vi "Curvature of Bezier Curve.vi"(11 "curve":T1) -> (3 "curvature":dbl[](array[numeric]))   [LabVIEW 2019]
uses:
  Types/Bezier Curve.ctl
panel:
  in  "percision":dbl
  in  "ctrl points":cluster{dbl, dbl}[](array[cluster])
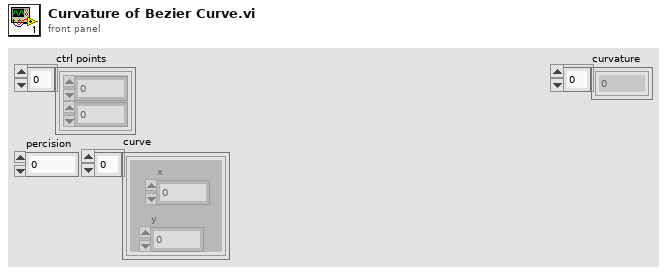
[diagram p1: front panel]
types:
  T1 = typedef "Bezier Curve.ctl" = cluster{"x":dbl, "y":dbl}[]
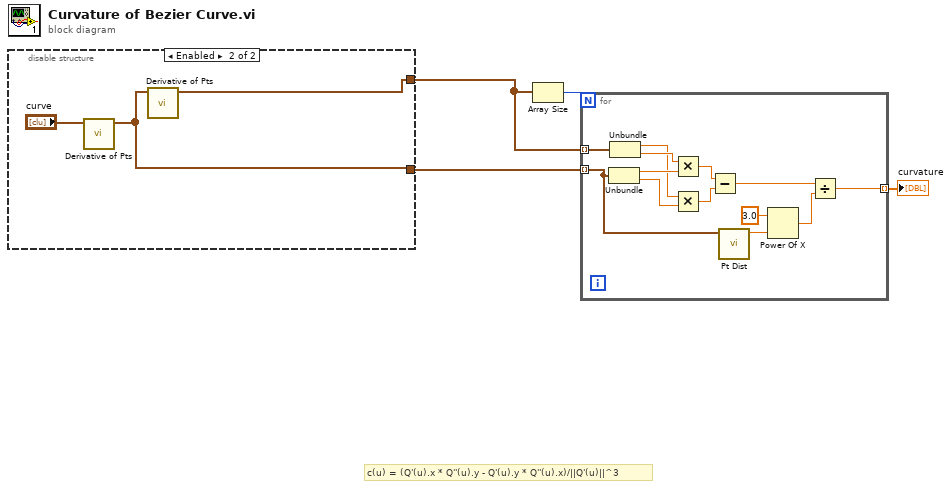
[diagram p0: block diagram]
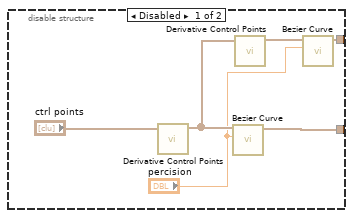
[diagram p2: hidden frame]
diagram:
  # "c(u) = (Q'(u).x * Q''(u).y - Q'(u).y * Q''(u).x)/||Q'(u)||^3"
  n1 = disable-structure shown="Enabled" {
    disable-tunnel: [w6 w12] -> w3
    disable-tunnel: [w5 w11] -> w2
    frame Disabled {
      n2 = call "Derivative Control Points.vi"("ctrl points"="ctrl points") -> ("d ctrl pts"=w9:cluster{dbl, dbl}[])  [unwired: 10 in]
      n3 = call "Bezier Curve.vi"("percision"="percision", "ctrl points"=w9) -> ("curve"=w5:T1)  [unwired: 9 in]
      n4 = call "Derivative Control Points.vi"("ctrl points"=w9) -> ("d ctrl pts"=w8:cluster{dbl, dbl}[])  [unwired: 10 in]
      n5 = call "Bezier Curve.vi"("percision"="percision", "ctrl points"=w8) -> ("curve"=w6:T1)  [unwired: 9 in]
    }
    frame Enabled {
      n6 = call "Derivative of Pts.vi"("pts"="curve") -> ("pts out"=w11:cluster{dbl, dbl}[])  [unwired: 10 in]
      n7 = call "Derivative of Pts.vi"("pts"=w11) -> ("pts out"=w12:cluster{dbl, dbl}[])  [unwired: 10 in]
    }
  }
  n8 = Array Size(array=w3) -> (size(s)=w4:i32)
  n9 = for {
    N: w4 -> [_]
    tunnel: w3 -> [w26] mode=indexing
    tunnel: w2 -> [w18] mode=indexing
    tunnel: [w14] -> w1 mode=indexing
    n10 = Unbundle(w18) -> (w25:dbl, w22:dbl)
    n11 = Unbundle(w26) -> (w23:dbl, w24:dbl)
    n12 = Multiply(x=w24, y=w25) -> (x*y=w20:dbl)
    n13 = Multiply(x=w23, y=w22) -> (x*y=w21:dbl)
    n14 = Subtract(x=w20, y=w21) -> (x-y=w19:dbl)
    n15 = call "Pt Dist.vi"("point a"=w18) -> ("dist"=w17:dbl)  [unwired: 10 in]
    n16 = Power Of X(1:w17, 2:3.0 ("y")) -> (0:w15:dbl)
    n17 = Divide(x=w19, y=w15) -> (x/y=w14:dbl)
  }
  "curvature" <- w1
